vi "Accurate Measure With Setting_ver2_2.vi"(0 "DMM ref in":refnum<visa-resource-name>, 1 "Accurate Measure Setting":T1={"Enable DMM Relay"=FALSE, "Measure Current Only"=FALSE, [], "channel_count"=11}, 2 "P_current_count":i32, 3 "N_current_count":i32, 5 "DMM error in":errorcluster, 7 "Current Sense \nResitance Array":dbl[](array[numeric])=[1.0032214, 1.00250644, 1.00234822, 1.0040944, 1.0017711, 1.00229431, 1.00344206, 1.00482066, 1.00381056, 1.00290978, 1.00333016, 1.00367587], 9 "ESP32 ref in":refnum<visa-resource-name>, 11 "ESP32 error in":errorcluster, 12 "current_mode":u8[](array[numeric])=[0, 0, 0, 0, 0, 0, 0, 0, 0, 0, 0]) -> (4 "DMM ref out":refnum<visa-resource-name>, 6 "DMM error out":errorcluster, 8 "Accurate Data":dbl[](array[numeric]), 10 "ESP32 ref out":refnum<visa-resource-name>, 13 "time_out_count":i32, 14 "Standard Deviation of Data":dbl[](array[numeric]), 15 "ESP32 error out":errorcluster)   [LabVIEW 2023]
uses:
  <instrlib>/Agilent 3446X Series/Agilent 3446X Series.lvlib
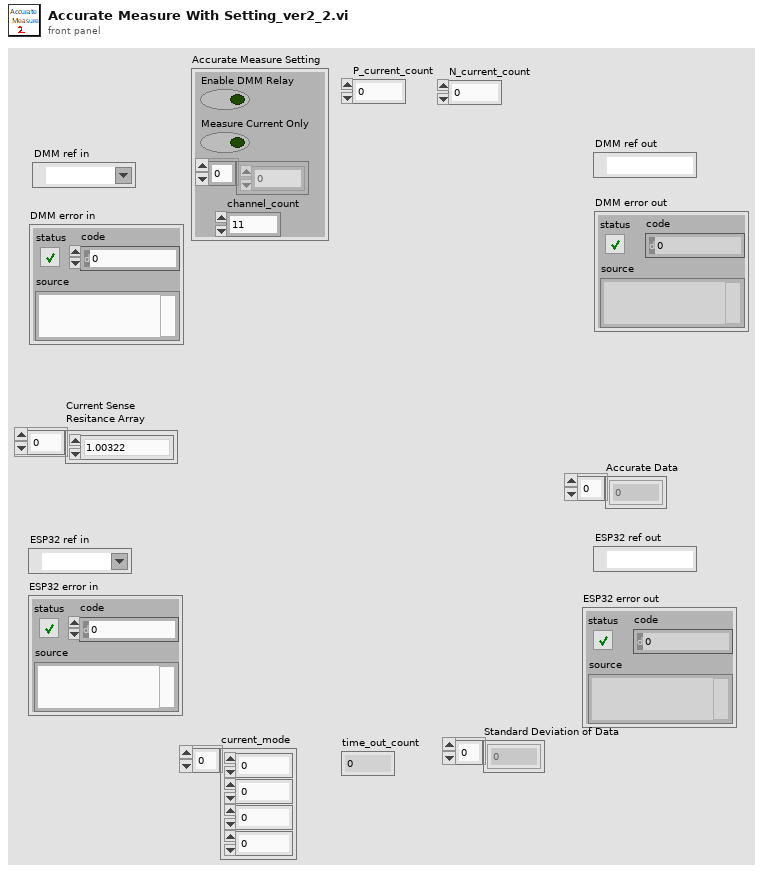
[diagram p1: front panel]
types:
  T1 = cluster{"Enable DMM Relay":bool, "Measure Current Only":bool, dbl[], "channel_count":i32}
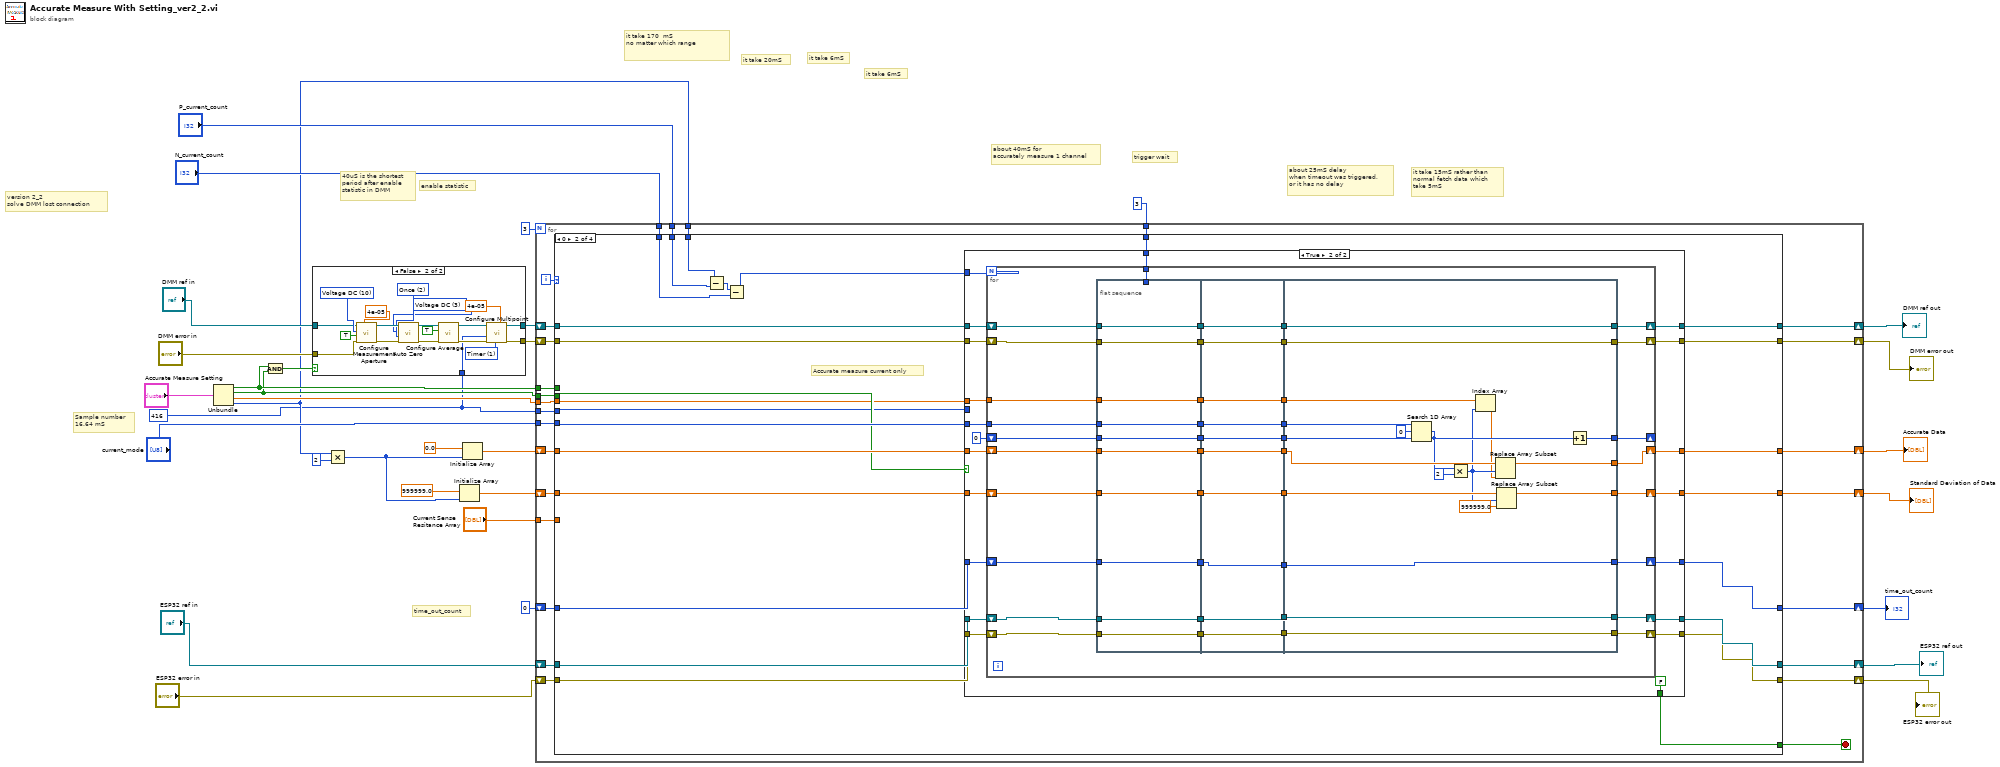
[diagram p0: block diagram]
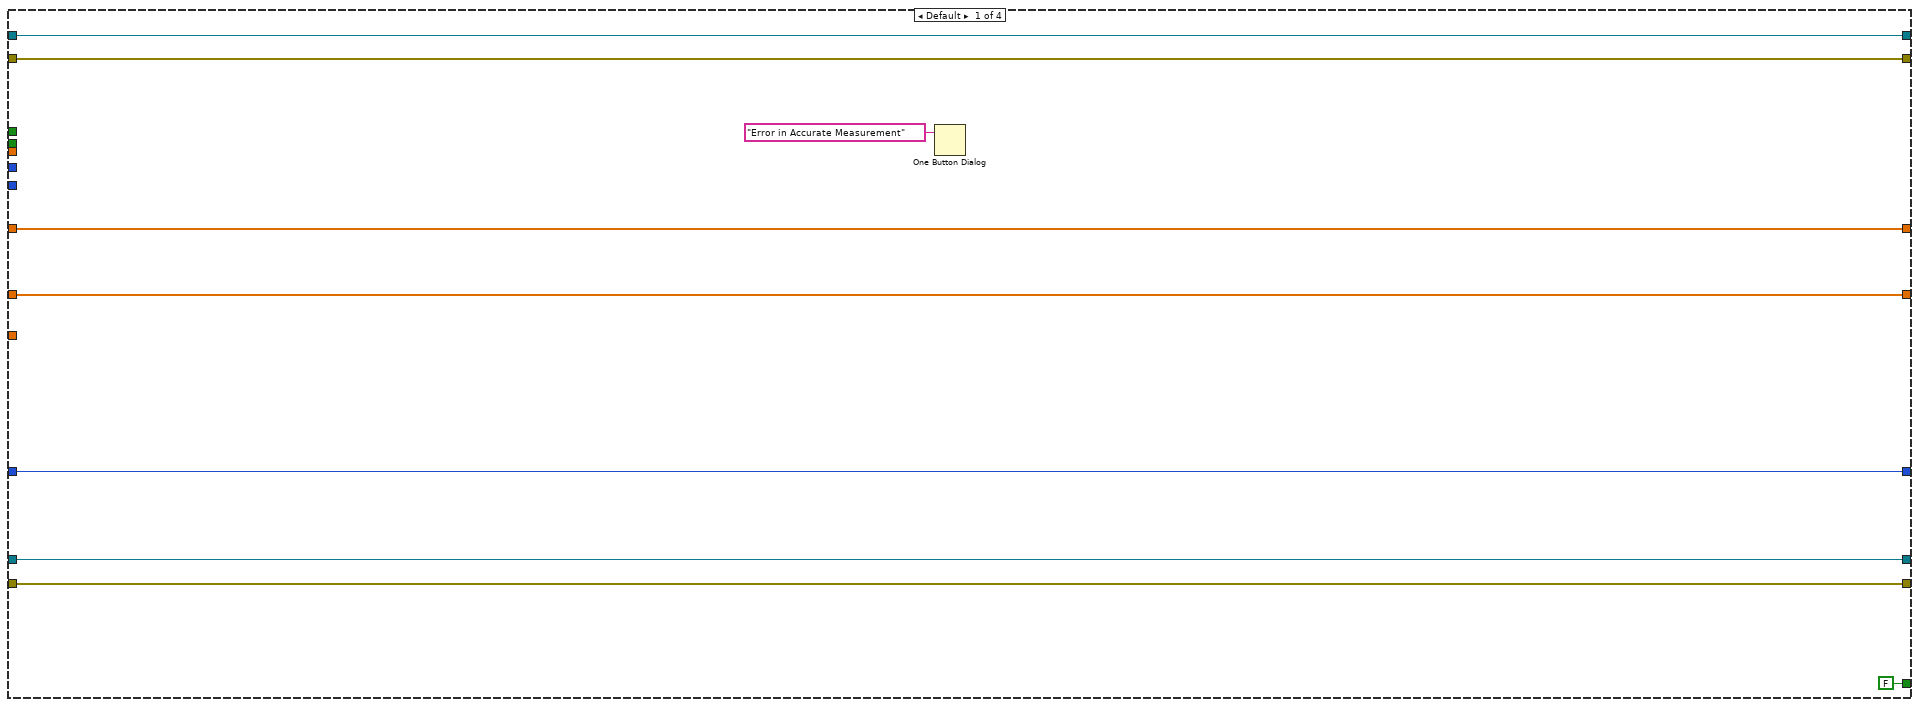
[diagram p3: hidden frame]
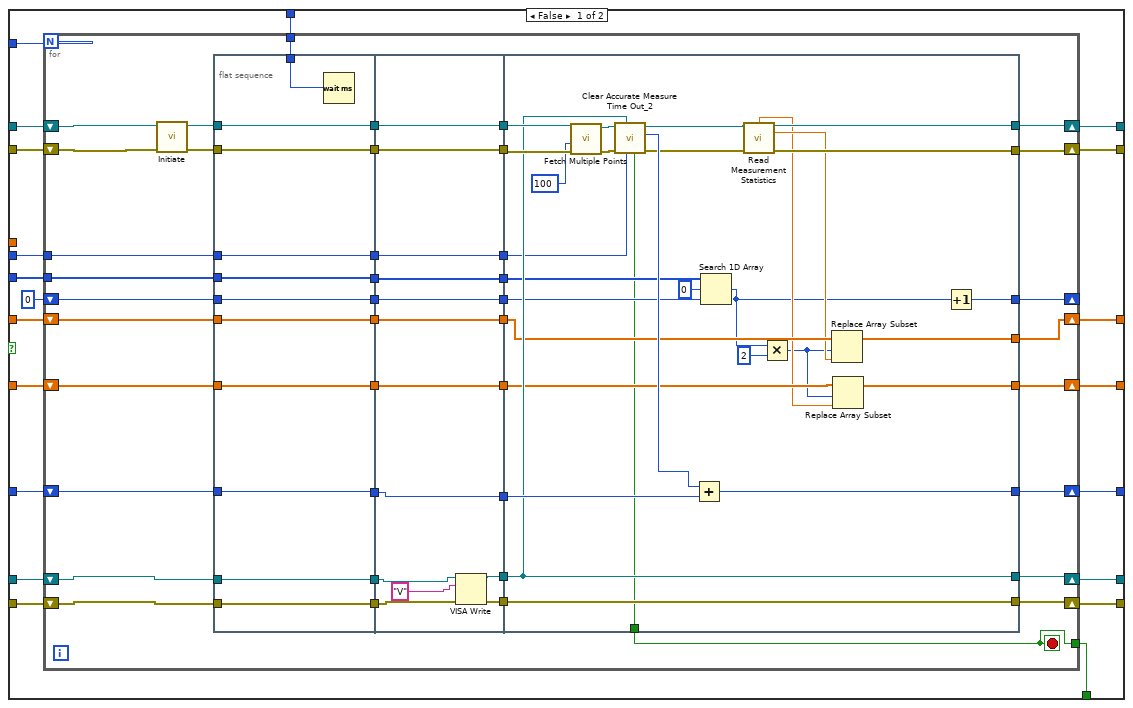
[diagram p4: hidden frame]
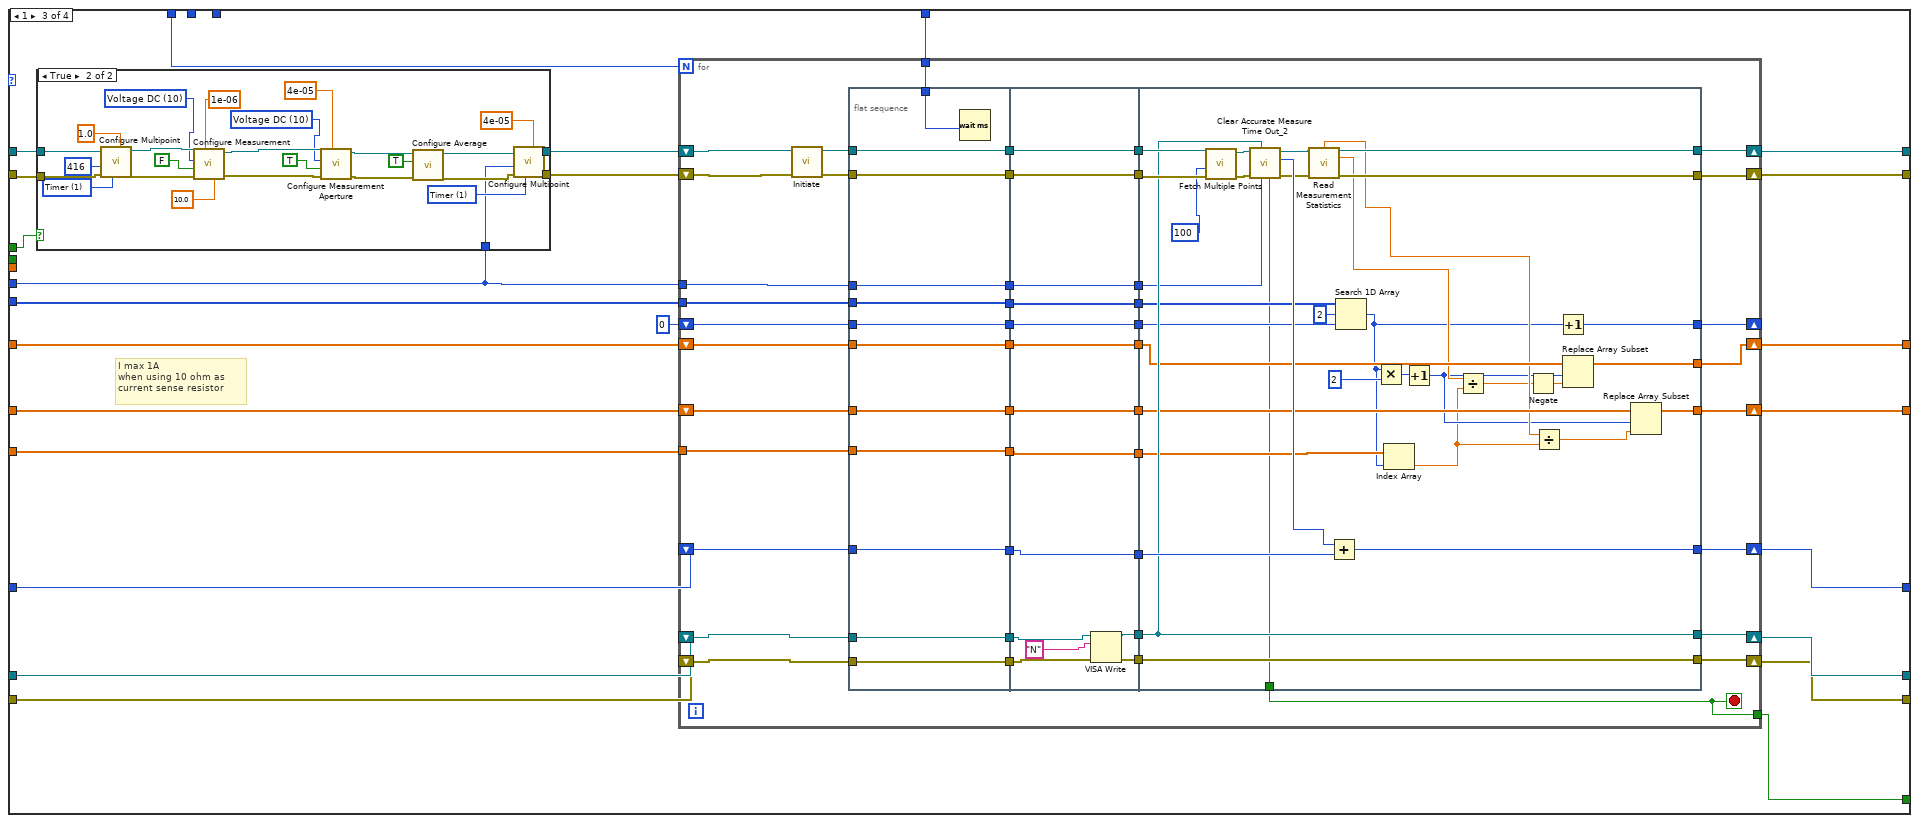
[diagram p5: hidden frame]
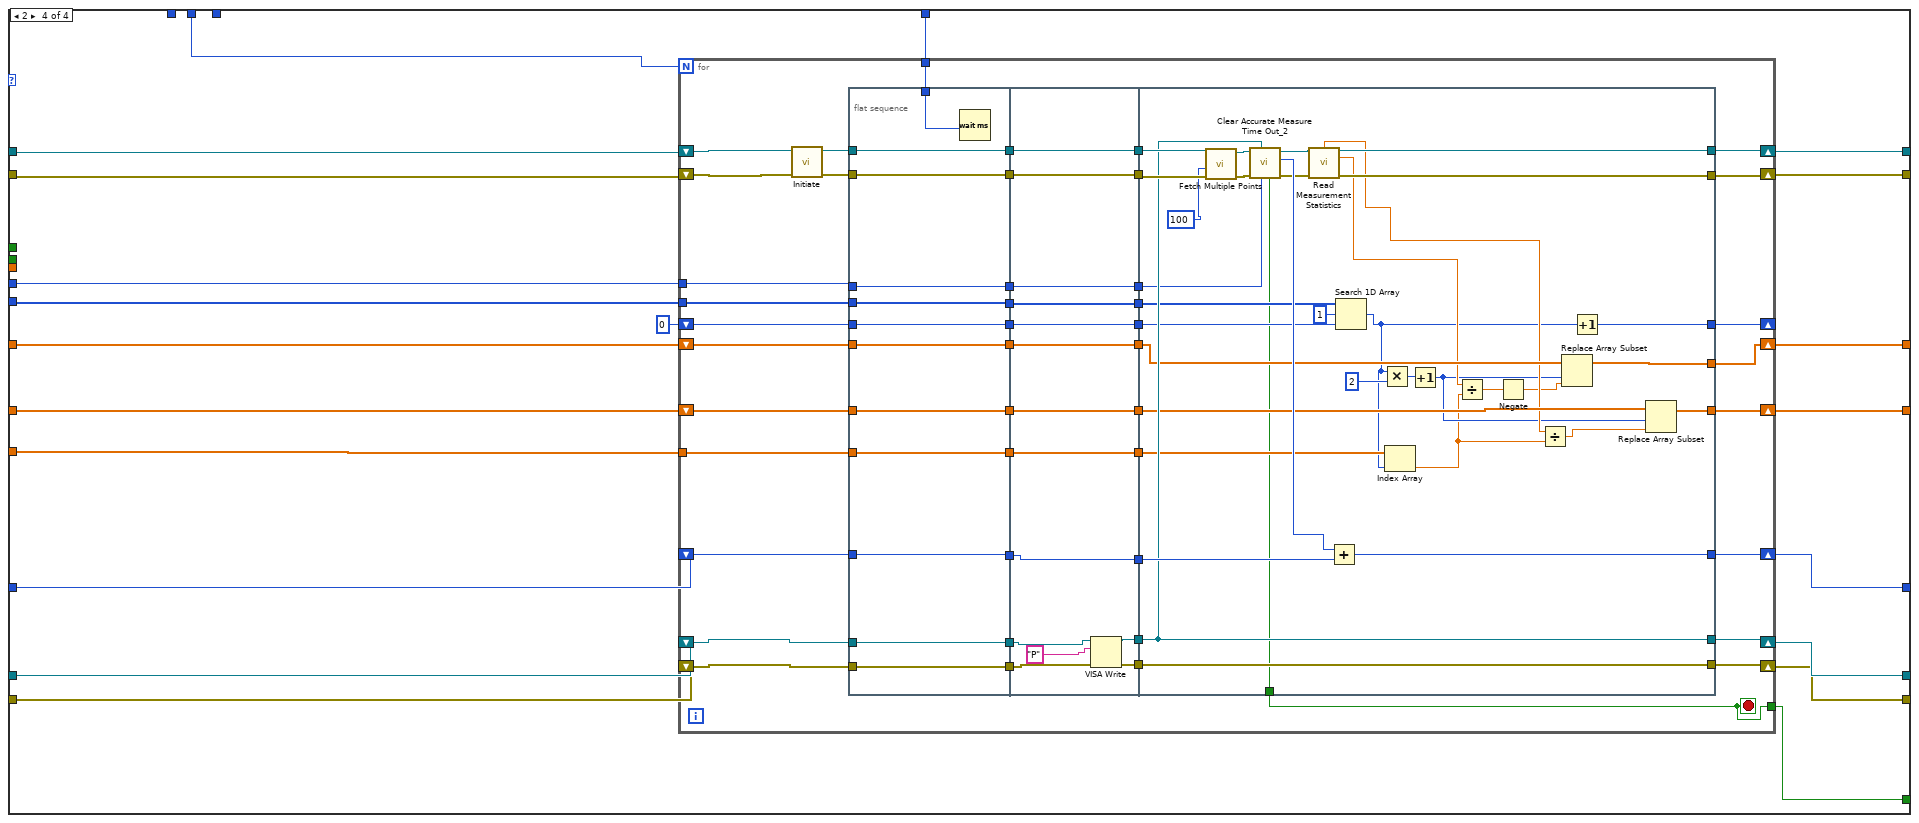
[diagram p7: hidden frame]
diagram:
  w1 = 416 ("Sample Count (1)")
  # "version 2_2\nsolve DMM lost connection"
  # "it take 6mS"
  # "it take 6mS"
  # "it take 20mS"
  # "it take 170  mS\nno matter which range"
  # "it take 15mS rather than\nnormal fetch data which \ntake 5mS"
  # "about 40mS for \naccurately measure 1 channel"
  # "about 25mS delay\nwhen timeout was triggered,\nor it has no delay"
  # "time_out_count"
  # "trigger wait"
  # "Sample number\n16.64 mS"
  # "enable statistic"
  # "40uS is the shortest\nperiod after enable \nstatistic in DMM"
  n1 = Unbundle("Accurate Measure Setting") -> ("Enable DMM Relay"=w6:bool, "Measure Current Only"=w5:bool, w7:dbl[], "channel_count"=w3:i32)
  n2 = And(x=w6, y=w5) -> (x .and. y?=w4:bool)
  n3 = case shown="False" w4 {
    tunnel: [w35 w40] -> w33
    tunnel: [w34 w39] -> w32
    tunnel: "DMM ref in" -> [w35 w38]
    tunnel: "DMM error in" -> [w34 w37]
    tunnel: w1 -> [_ w36]
    frame True {
    }
    frame False {
      w41 = 1 items=["Immediate", "Timer"] ("Sample Source (0: Immediate)")
      w48 = 3 items=["Current DC", "Resistance", "Temperature", "Voltage DC"] ("Zero Type (0: Current DC)")
      w49 = 2 items=["Disable", "Enable", "Once"] ("Auto Zero (1: Enable)")
      w45 = 10 items=["Continuity", "Current AC", "Current DC", "Diode", "Frequency", "Resistance 4-wire", "Period", "Resistance 2-wire", "Temperature", "Voltage AC", "Voltage DC", "Voltage DC Ratio", "Capacitance"] ("Measurement Function (0: Continuity)")
      n4 = call <instrlib>:"Configure Measurement Aperture.vi"("Aperture Time (0.1s)"=4e-05, "error in (no error)"=w37, "Enable Aperture (F: Disable)"=TRUE, "Measurement Function (0: Continuity)"=w45, "VISA resource name"=w38) -> ("error out"=w52:errorcluster, "VISA resource name out"=w51:refnum<visa-resource-name>)  [unwired: 5 in]
      n5 = call <instrlib>:"Auto Zero.vi"("error in (no error)"=w52, "Auto Zero (1: Enable)"=w49, "Zero Type (0: Current DC)"=w48, "VISA resource name"=w51) -> ("error out"=w54:errorcluster, "VISA resource name out"=w53:refnum<visa-resource-name>)  [unwired: 6 in]
      n6 = call <instrlib>:"Configure Average.vi"("error in (no error)"=w54, "Enable Statistics (F: Disable)"=TRUE, "VISA resource name"=w53) -> ("error out"=w43:errorcluster, "VISA resource name out"=w44:refnum<visa-resource-name>)  [unwired: 7 in]
      n7 = call <instrlib>:"Configure Multipoint.vi"("Sample Interval (1 Second)"=4e-05, "Sample Source (0: Immediate)"=w41, "error in (no error)"=w43, "Sample Count (1)"=w36, "VISA resource name"=w44) -> ("error out"=w39:errorcluster, "VISA resource name out"=w40:refnum<visa-resource-name>)  [unwired: 2 in, 3 out]
    }
  }
  n8 = Multiply(x=w3, y=2) -> (x*y=w9:i32)
  n9 = Initialize Array(999999.0 ("Arithmetic Mean"), w9) -> (w18:dbl[])
  n10 = Initialize Array(0.0 ("Arithmetic Mean"), w9) -> (w21:dbl[])
  n11 = for {
    N: 3 -> [_]
    shift-right: [w78] -> w14
    shift-left: "ESP32 ref in" -> [w80]
    shift-right: [w77] -> w13
    shift-left: "ESP32 error in" -> [w79]
    shift-right: [w74] -> w16
    shift-left: w33 -> [w76]
    shift-right: [w73] -> w15
    shift-left: w32 -> [w75]
    tunnel: w3 -> [w72]
    tunnel: "P_current_count" -> [w71]
    tunnel: "N_current_count" -> [w70]
    tunnel: u32 3 ("milliseconds to wait") -> [w69]
    shift-right: [w68] -> w23
    shift-left: 0 -> [w67]
    shift-right: [w61] -> w12
    shift-left: w21 -> [w66]
    tunnel: "current_mode" -> [w65]
    shift-right: [w62] -> w11
    shift-left: w18 -> [w63]
    tunnel: w6 -> [w60]
    tunnel: w5 -> [w59]
    tunnel: w7 -> [w58]
    tunnel: "Current Sense \nResitance Array" -> [w57]
    tunnel: w1 -> [w56]
    i -> [w64]
    stop <- w55 stop-if-true
    n12 = case shown="0" w64 {
      tunnel: w80 -> [w87 w110 w351 w506]
      tunnel: w79 -> [w86 w109 w350 w505]
      tunnel: [w87 w106 w347 w502] -> w78
      tunnel: [w86 w105 w346 w501] -> w77
      tunnel: w76 -> [w89 w112 w336 w491]
      tunnel: w75 -> [w88 w111 w335 w490]
      tunnel: [w89 w108 w349 w504] -> w74
      tunnel: [w88 w107 w348 w503] -> w73
      tunnel: w72 -> [_ w104 _ _]
      tunnel: w71 -> [_ w103 _ w488]
      tunnel: w70 -> [_ w102 w330 _]
      tunnel: [w83 w100 w344 w499] -> w68
      tunnel: w69 -> [_ w101 w345 w500]
      tunnel: w67 -> [w83 w99 w343 w498]
      tunnel: w66 -> [w85 w97 w341 w496]
      tunnel: w65 -> [_ w98 w342 w497]
      tunnel: w63 -> [w84 w96 w339 w494]
      tunnel: [w84 w95 w338 w493] -> w62
      tunnel: [w85 w94 w337 w492] -> w61
      tunnel: w60 -> [_ _ w332 _]
      tunnel: w59 -> [_ w93 _ _]
      tunnel: w58 -> [_ w92 _ _]
      tunnel: w57 -> [_ _ w331 w489]
      tunnel: w56 -> [_ w91 w329 w487]
      tunnel: [FALSE ("lost connection") w90 w328 w486] -> w55
      frame Default {
        n13 = One Button Dialog(message="Error in Accurate Measurement") -> ()  [unwired: 1 in, 1 out]
      }
      frame 0 {
        # "Accurate measure current only"
        n14 = Subtract(x=w104, y=w103) -> (x-y=w114:i32)
        n15 = Subtract(x=w114, y=w102) -> (x-y=w113:i32)
        n16 = case shown="True" w93 {
          tunnel: w113 -> [w134 w249]
          tunnel: w112 -> [w133 w248]
          tunnel: w111 -> [w132 w247]
          tunnel: w110 -> [w131 w246]
          tunnel: w109 -> [w130 w245]
          tunnel: [w129 w244] -> w108
          tunnel: [w128 w243] -> w107
          tunnel: [w127 w242] -> w106
          tunnel: [w126 w241] -> w105
          tunnel: w101 -> [w125 w240]
          tunnel: [w124 w239] -> w100
          tunnel: w99 -> [w123 w238]
          tunnel: w98 -> [w122 w237]
          tunnel: w97 -> [w121 w236]
          tunnel: w96 -> [w119 w234]
          tunnel: [w118 w233] -> w95
          tunnel: [w117 w232] -> w94
          tunnel: w92 -> [_ w231]
          tunnel: w91 -> [w116 _]
          tunnel: [w115 FALSE ("lost connection")] -> w90
          frame False {
            n17 = for {
              N: w134 -> [_]
              shift-right: [w172] -> w129
              shift-left: w133 -> [w176]
              shift-right: [w171] -> w128
              shift-left: w132 -> [w175]
              shift-right: [w170] -> w127
              shift-left: w131 -> [w174]
              shift-right: [w169] -> w126
              shift-left: w130 -> [w173]
              tunnel: w125 -> [w155]
              shift-right: [w154] -> w124
              shift-left: w123 -> [w168]
              tunnel: w122 -> [w152]
              shift-right: [w140] -> w117
              shift-left: w121 -> [w149]
              shift-right: [w144] -> _
              shift-left: 0 ("index of element") -> [w145]
              shift-right: [w139] -> w118
              shift-left: w119 -> [w142]
              tunnel: w116 -> [w136]
              tunnel: [w135] -> w115
              stop <- w135 stop-if-true
              n18 = call <instrlib>:"Initiate.vi"("error in (no error)"=w175, "VISA resource name"=w176) -> ("error out"=w156:errorcluster, "VISA resource name out"=w157:refnum<visa-resource-name>)  [unwired: 8 in]
              n19 = flat-sequence {
                tunnel: [w187] -> w167
                tunnel: w174 -> [w187]
                tunnel: [w186] -> w166
                tunnel: w173 -> [w186]
                tunnel: w157 -> [w185]
                tunnel: [w185] -> w165
                tunnel: [w184] -> w164
                tunnel: w156 -> [w184]
                tunnel: [w183] -> w163
                tunnel: w168 -> [w183]
                tunnel: w155 -> [w182]
                tunnel: [w181] -> w153
                tunnel: w152 -> [w181]
                tunnel: [w180] -> w150
                tunnel: w149 -> [w180]
                tunnel: w145 -> [w179]
                tunnel: [w179] -> w147
                tunnel: [w178] -> w143
                tunnel: w142 -> [w178]
                tunnel: w136 -> [w177]
                tunnel: [w177] -> w138
                tunnel: w167 -> [w200]
                tunnel: w166 -> [w199]
                tunnel: w165 -> [w198]
                tunnel: [w198] -> w159
                tunnel: w164 -> [w197]
                tunnel: [w197] -> w160
                tunnel: [w196] -> w161
                tunnel: [w195] -> w162
                tunnel: w163 -> [w193]
                tunnel: [w193] -> w158
                tunnel: w153 -> [w192]
                tunnel: [w192] -> w151
                tunnel: w150 -> [w191]
                tunnel: [w191] -> w148
                tunnel: w147 -> [w190]
                tunnel: [w190] -> w146
                tunnel: w143 -> [w189]
                tunnel: [w189] -> w141
                tunnel: w138 -> [w188]
                tunnel: [w188] -> w137
                tunnel: [w229] -> w169
                tunnel: [w217] -> w170
                tunnel: [w221] -> w171
                tunnel: [w222] -> w172
                tunnel: w162 -> [w229]
                tunnel: w161 -> [w217]
                tunnel: w160 -> [w228]
                tunnel: w159 -> [w227]
                tunnel: [w223] -> w154
                tunnel: w158 -> [w218]
                tunnel: w151 -> [w216]
                tunnel: w148 -> [w212]
                tunnel: w146 -> [w214]
                tunnel: [w213] -> w144
                tunnel: w141 -> [w210]
                tunnel: [w208] -> w140
                tunnel: [w207] -> w139
                tunnel: w137 -> [w202]
                tunnel: [w201] -> w135
                frame #0 {
                  n20 = Wait (ms)(milliseconds to wait=w182) -> ()  [unwired: 1 out]
                }
                frame #1 {
                  n21 = VISA Write(VISA resource name=w200, write buffer="V" ("data in"), error in (no error)=w199) -> (VISA resource name out=w196:refnum<visa-resource-name>, error out=w195:errorcluster)  [unwired: 1 out]
                }
                frame #2 {
                  n22 = call <instrlib>:"Fetch Multiple Points.vi"("error in (no error)"=w228, "Timeout (10000 ms)"=100, "VISA resource name"=w227) -> ("error out"=w225:errorcluster, "VISA resource name out"=w226:refnum<visa-resource-name>)  [unwired: 1 in, 6 out]
                  n23 = call "Clear Accurate Measure Time Out_2.vi"("Sample Count (1)"=w202, "ESP32 ref"=w217, "error in (no error)"=w225, "DMM ref"=w226) -> ("error out"=w219:errorcluster, "Time out count"=w224:i32, "VISA Refnum out"=w220:refnum<visa-resource-name>, "lost connection"=w201:bool)  [unwired: 3 in, 1 out]
                  n24 = Add(x=w224, y=w218) -> (x+y=w223:i32)
                  n25 = Search 1D Array(1D array=w216, element=u8 0, start index (0)=w214) -> (index of element=w205:i32)
                  n26 = call <instrlib>:"Read Measurement Statistics.vi"("VISA resource name"=w220, "error in (no error)"=w219) -> ("Standard Deviation"=w209:dbl, "VISA resource name out"=w222:refnum<visa-resource-name>, "Arithmetic Mean"=w211:dbl, "error out"=w221:errorcluster)  [unwired: 6 in, 4 out]
                  n27 = Multiply(x=w205, y=2) -> (x*y=w203:i32)
                  n28 = Replace Array Subset(array=w212, new element=w211, index=w203) -> (w208:dbl[])
                  n29 = Replace Array Subset(array=w210, new element=w209, index=w203) -> (w207:dbl[])
                  n30 = Increment(x=w205) -> (x+1=w213:i32)
                }
              }
            }
          }
          frame True {
            n31 = for {
              N: w249 -> [_]
              shift-right: [w258] -> w244
              shift-left: w248 -> [w260]
              shift-right: [w253] -> w243
              shift-left: w247 -> [w255]
              shift-right: [w286] -> w242
              shift-left: w246 -> [w288]
              shift-right: [w285] -> w241
              shift-left: w245 -> [w287]
              tunnel: w240 -> [w277]
              shift-right: [w276] -> w239
              shift-left: w238 -> [w284]
              tunnel: w237 -> [w274]
              shift-right: [w262] -> w232
              shift-left: w236 -> [w271]
              shift-right: [w266] -> _
              shift-left: 0 ("index of element") -> [w267]
              shift-right: [w261] -> w233
              shift-left: w234 -> [w264]
              tunnel: w231 -> [w250]
              n32 = flat-sequence {
                tunnel: [w298] -> w283
                tunnel: w288 -> [w298]
                tunnel: [w297] -> w282
                tunnel: w287 -> [w297]
                tunnel: [w296] -> w281
                tunnel: w284 -> [w296]
                tunnel: w277 -> [_]
                tunnel: [w295] -> w275
                tunnel: w274 -> [w295]
                tunnel: [w294] -> w272
                tunnel: w271 -> [w294]
                tunnel: w267 -> [w293]
                tunnel: [w293] -> w269
                tunnel: [w292] -> w265
                tunnel: w264 -> [w292]
                tunnel: w260 -> [w291]
                tunnel: [w291] -> w257
                tunnel: [w290] -> w256
                tunnel: w255 -> [w290]
                tunnel: [w289] -> w252
                tunnel: w250 -> [w289]
                tunnel: w283 -> [w301]
                tunnel: w282 -> [w300]
                tunnel: [w301] -> w279
                tunnel: [w300] -> w280
                tunnel: w281 -> [w308]
                tunnel: [w308] -> w278
                tunnel: w275 -> [w307]
                tunnel: [w307] -> w273
                tunnel: w272 -> [w306]
                tunnel: [w306] -> w270
                tunnel: w269 -> [w305]
                tunnel: [w305] -> w268
                tunnel: w265 -> [w304]
                tunnel: [w304] -> w263
                tunnel: [w303] -> w259
                tunnel: w257 -> [w303]
                tunnel: w256 -> [w302]
                tunnel: [w302] -> w254
                tunnel: w252 -> [w299]
                tunnel: [w299] -> w251
                tunnel: [w327] -> w285
                tunnel: [w326] -> w286
                tunnel: w280 -> [w327]
                tunnel: w279 -> [w326]
                tunnel: [w309] -> w276
                tunnel: w278 -> [w309]
                tunnel: w273 -> [w325]
                tunnel: w270 -> [w321]
                tunnel: w268 -> [w323]
                tunnel: [w322] -> w266
                tunnel: w263 -> [w320]
                tunnel: [w319] -> w262
                tunnel: [w318] -> w261
                tunnel: w259 -> [w315]
                tunnel: [w315] -> w258
                tunnel: [w314] -> w253
                tunnel: w254 -> [w314]
                tunnel: w251 -> [w312]
                frame #0 {
                }
                frame #1 {
                }
                frame #2 {
                  n33 = Search 1D Array(1D array=w325, element=u8 0, start index (0)=w323) -> (index of element=w317:i32)
                  n34 = Multiply(x=w317, y=2) -> (x*y=w311:i32)
                  n35 = Index Array(array=w312, index=w311) -> (element=w310:dbl)
                  n36 = Replace Array Subset(array=w321, new element=w310, index=w311) -> (w319:dbl[])
                  n37 = Replace Array Subset(array=w320, new element=999999.0 ("new element/subarray"), index=w311) -> (w318:dbl[])
                  n38 = Increment(x=w317) -> (x+1=w322:i32)
                }
              }
            }
          }
        }
      }
      frame 1 {
        # "I max 1A\nwhen using 10 ohm as \ncurrent sense resistor"
        n39 = case shown="True" w332 {
          tunnel: w336 -> [w353 w360]
          tunnel: w335 -> [w352 w359]
          tunnel: [w353 w358] -> w334
          tunnel: [w352 w357] -> w333
          tunnel: w329 -> [_ w354]
          frame False {
          }
          frame True {
            w369 = 1 items=["Immediate", "Timer"] ("Sample Source (0: Immediate)")
            w366 = 10 items=["Continuity", "Current AC", "Current DC", "Diode", "Frequency", "Resistance 4-wire", "Period", "Resistance 2-wire", "Temperature", "Voltage AC", "Voltage DC", "Voltage DC Ratio", "Capacitance"] ("Measurement Function (0: Continuity)")
            w364 = 1 items=["Immediate", "Timer"] ("Sample Source (0: Immediate)")
            w361 = 10 items=["Continuity", "Current AC", "Current DC", "Diode", "Frequency", "Resistance 4-wire", "Period", "Resistance 2-wire", "Temperature", "Voltage AC", "Voltage DC", "Voltage DC Ratio", "Capacitance"] ("Measurement Function (10: Voltage DC)")
            n40 = call <instrlib>:"Configure Multipoint.vi"("Sample Interval (1 Second)"=1.0, "Sample Source (0: Immediate)"=w364, "error in (no error)"=w359, "Sample Count (1)"=416, "VISA resource name"=w360) -> ("error out"=w376:errorcluster, "VISA resource name out"=w375:refnum<visa-resource-name>)  [unwired: 2 in, 3 out]
            n41 = call <instrlib>:"Configure Measurement.vi"("Manual Range (1)"=10.0, "Absolute Resolution (1E-6)"=1e-06 ("x"), "error in (no error)"=w376, "Auto Range (T: Enable)"=FALSE, "Measurement Function (10: Voltage DC)"=w361, "VISA resource name"=w375) -> ("error out"=w373:errorcluster, "VISA resource name out"=w374:refnum<visa-resource-name>)  [unwired: 4 out]
            n42 = call <instrlib>:"Configure Measurement Aperture.vi"("Aperture Time (0.1s)"=4e-05, "error in (no error)"=w373, "Enable Aperture (F: Disable)"=TRUE, "Measurement Function (0: Continuity)"=w366, "VISA resource name"=w374) -> ("error out"=w378:errorcluster, "VISA resource name out"=w379:refnum<visa-resource-name>)  [unwired: 5 in]
            n43 = call <instrlib>:"Configure Average.vi"("error in (no error)"=w378, "Enable Statistics (F: Disable)"=TRUE, "VISA resource name"=w379) -> ("error out"=w377:errorcluster, "VISA resource name out"=w372:refnum<visa-resource-name>)  [unwired: 7 in]
            n44 = call <instrlib>:"Configure Multipoint.vi"("Sample Interval (1 Second)"=4e-05, "Sample Source (0: Immediate)"=w369, "error in (no error)"=w377, "Sample Count (1)"=w354, "VISA resource name"=w372) -> ("error out"=w357:errorcluster, "VISA resource name out"=w358:refnum<visa-resource-name>)  [unwired: 2 in, 3 out]
          }
        }
        n45 = for {
          N: w330 -> [_]
          shift-right: [w420] -> w349
          shift-left: w334 -> [w424]
          shift-right: [w419] -> w348
          shift-left: w333 -> [w423]
          shift-right: [w418] -> w347
          shift-left: w351 -> [w422]
          shift-right: [w417] -> w346
          shift-left: w350 -> [w421]
          tunnel: w345 -> [w403]
          shift-right: [w402] -> w344
          shift-left: w343 -> [w416]
          tunnel: w342 -> [w400]
          shift-right: [w388] -> w337
          shift-left: w341 -> [w397]
          shift-right: [w392] -> _
          shift-left: 0 ("index of element") -> [w393]
          shift-right: [w387] -> w338
          shift-left: w339 -> [w390]
          tunnel: w331 -> [w385]
          tunnel: w329 -> [w383]
          tunnel: [w380] -> w328
          stop <- w380 stop-if-true
          n46 = call <instrlib>:"Initiate.vi"("error in (no error)"=w423, "VISA resource name"=w424) -> ("error out"=w404:errorcluster, "VISA resource name out"=w405:refnum<visa-resource-name>)  [unwired: 8 in]
          n47 = flat-sequence {
            tunnel: [w436] -> w415
            tunnel: w422 -> [w436]
            tunnel: [w435] -> w414
            tunnel: w421 -> [w435]
            tunnel: w405 -> [w434]
            tunnel: [w434] -> w413
            tunnel: [w433] -> w412
            tunnel: w404 -> [w433]
            tunnel: [w432] -> w411
            tunnel: w416 -> [w432]
            tunnel: w403 -> [w431]
            tunnel: [w430] -> w401
            tunnel: w400 -> [w430]
            tunnel: [w429] -> w398
            tunnel: w397 -> [w429]
            tunnel: w393 -> [w428]
            tunnel: [w428] -> w395
            tunnel: [w427] -> w391
            tunnel: w390 -> [w427]
            tunnel: [w426] -> w386
            tunnel: w385 -> [w426]
            tunnel: w383 -> [w425]
            tunnel: [w425] -> w382
            tunnel: w415 -> [w450]
            tunnel: w414 -> [w449]
            tunnel: w413 -> [w448]
            tunnel: [w448] -> w407
            tunnel: w412 -> [w447]
            tunnel: [w447] -> w408
            tunnel: [w446] -> w409
            tunnel: [w445] -> w410
            tunnel: w411 -> [w443]
            tunnel: [w443] -> w406
            tunnel: w401 -> [w442]
            tunnel: [w442] -> w399
            tunnel: w398 -> [w441]
            tunnel: [w441] -> w396
            tunnel: w395 -> [w440]
            tunnel: [w440] -> w394
            tunnel: w391 -> [w439]
            tunnel: [w439] -> w389
            tunnel: w386 -> [w438]
            tunnel: [w438] -> w384
            tunnel: w382 -> [w437]
            tunnel: [w437] -> w381
            tunnel: [w485] -> w417
            tunnel: [w473] -> w418
            tunnel: [w477] -> w419
            tunnel: [w478] -> w420
            tunnel: w410 -> [w485]
            tunnel: w409 -> [w473]
            tunnel: w408 -> [w484]
            tunnel: w407 -> [w483]
            tunnel: [w479] -> w402
            tunnel: w406 -> [w474]
            tunnel: w399 -> [w472]
            tunnel: w396 -> [w469]
            tunnel: w394 -> [w471]
            tunnel: [w470] -> w392
            tunnel: w389 -> [w468]
            tunnel: [w467] -> w388
            tunnel: [w466] -> w387
            tunnel: w384 -> [w462]
            tunnel: w381 -> [w452]
            tunnel: [w451] -> w380
            frame #0 {
              n48 = Wait (ms)(milliseconds to wait=w431) -> ()  [unwired: 1 out]
            }
            frame #1 {
              n49 = VISA Write(VISA resource name=w450, write buffer="N" ("data in"), error in (no error)=w449) -> (VISA resource name out=w446:refnum<visa-resource-name>, error out=w445:errorcluster)  [unwired: 1 out]
            }
            frame #2 {
              n50 = call <instrlib>:"Fetch Multiple Points.vi"("error in (no error)"=w484, "Timeout (10000 ms)"=100, "VISA resource name"=w483) -> ("error out"=w481:errorcluster, "VISA resource name out"=w482:refnum<visa-resource-name>)  [unwired: 1 in, 6 out]
              n51 = call "Clear Accurate Measure Time Out_2.vi"("Sample Count (1)"=w452, "ESP32 ref"=w473, "error in (no error)"=w481, "DMM ref"=w482) -> ("error out"=w475:errorcluster, "Time out count"=w480:i32, "VISA Refnum out"=w476:refnum<visa-resource-name>, "lost connection"=w451:bool)  [unwired: 3 in, 1 out]
              n52 = call <instrlib>:"Read Measurement Statistics.vi"("VISA resource name"=w476, "error in (no error)"=w475) -> ("Standard Deviation"=w464:dbl, "VISA resource name out"=w478:refnum<visa-resource-name>, "Arithmetic Mean"=w465:dbl, "error out"=w477:errorcluster)  [unwired: 6 in, 4 out]
              n53 = Add(x=w480, y=w474) -> (x+y=w479:i32)
              n54 = Search 1D Array(1D array=w472, element=u8 2, start index (0)=w471) -> (index of element=w457:i32)
              n55 = Multiply(x=w457, y=2) -> (x*y=w459:i32)
              n56 = Index Array(array=w462, index=w457) -> (element=w455:dbl)
              n57 = Increment(x=w459) -> (x+1=w458:i32)
              n58 = Divide(x=w465, y=w455) -> (x/y=w456:dbl)
              n59 = Negate(x=w456) -> (-x=w453:dbl)
              n60 = Divide(x=w464, y=w455) -> (x/y=w454:dbl)
              n61 = Increment(x=w457) -> (x+1=w470:i32)
              n62 = Replace Array Subset(array=w469, new element=w453, index=w458) -> (w467:dbl[])
              n63 = Replace Array Subset(array=w468, new element=w454, index=w458) -> (w466:dbl[])
            }
          }
        }
      }
      frame 2 {
        n64 = for {
          N: w488 -> [_]
          shift-right: [w547] -> w504
          shift-left: w491 -> [w551]
          shift-right: [w546] -> w503
          shift-left: w490 -> [w550]
          shift-right: [w545] -> w502
          shift-left: w506 -> [w549]
          shift-right: [w544] -> w501
          shift-left: w505 -> [w548]
          tunnel: w500 -> [w530]
          shift-right: [w529] -> w499
          shift-left: w498 -> [w543]
          tunnel: w497 -> [w527]
          shift-right: [w515] -> w492
          shift-left: w496 -> [w524]
          shift-right: [w519] -> _
          shift-left: 0 ("index of element") -> [w520]
          shift-right: [w514] -> w493
          shift-left: w494 -> [w517]
          tunnel: w489 -> [w512]
          tunnel: w487 -> [w508]
          tunnel: [w507] -> w486
          stop <- w507 stop-if-true
          n65 = call <instrlib>:"Initiate.vi"("error in (no error)"=w550, "VISA resource name"=w551) -> ("error out"=w531:errorcluster, "VISA resource name out"=w532:refnum<visa-resource-name>)  [unwired: 8 in]
          n66 = flat-sequence {
            tunnel: [w563] -> w542
            tunnel: w549 -> [w563]
            tunnel: [w562] -> w541
            tunnel: w548 -> [w562]
            tunnel: w532 -> [w561]
            tunnel: [w561] -> w540
            tunnel: [w560] -> w539
            tunnel: w531 -> [w560]
            tunnel: [w559] -> w538
            tunnel: w543 -> [w559]
            tunnel: w530 -> [w558]
            tunnel: [w557] -> w528
            tunnel: w527 -> [w557]
            tunnel: [w556] -> w525
            tunnel: w524 -> [w556]
            tunnel: w520 -> [w555]
            tunnel: [w555] -> w522
            tunnel: [w554] -> w518
            tunnel: w517 -> [w554]
            tunnel: [w553] -> w513
            tunnel: w512 -> [w553]
            tunnel: w508 -> [w552]
            tunnel: [w552] -> w510
            tunnel: w542 -> [w577]
            tunnel: w541 -> [w576]
            tunnel: w540 -> [w575]
            tunnel: [w575] -> w534
            tunnel: w539 -> [w574]
            tunnel: [w574] -> w535
            tunnel: [w573] -> w536
            tunnel: [w572] -> w537
            tunnel: w538 -> [w570]
            tunnel: [w570] -> w533
            tunnel: w528 -> [w569]
            tunnel: [w569] -> w526
            tunnel: w525 -> [w568]
            tunnel: [w568] -> w523
            tunnel: w522 -> [w567]
            tunnel: [w567] -> w521
            tunnel: w518 -> [w566]
            tunnel: [w566] -> w516
            tunnel: w513 -> [w565]
            tunnel: [w565] -> w511
            tunnel: w510 -> [w564]
            tunnel: [w564] -> w509
            tunnel: [w612] -> w544
            tunnel: [w600] -> w545
            tunnel: [w604] -> w546
            tunnel: [w605] -> w547
            tunnel: w537 -> [w612]
            tunnel: w536 -> [w600]
            tunnel: w535 -> [w611]
            tunnel: w534 -> [w610]
            tunnel: [w606] -> w529
            tunnel: w533 -> [w601]
            tunnel: w526 -> [w599]
            tunnel: w523 -> [w596]
            tunnel: w521 -> [w598]
            tunnel: [w597] -> w519
            tunnel: w516 -> [w595]
            tunnel: [w594] -> w515
            tunnel: [w593] -> w514
            tunnel: w511 -> [w589]
            tunnel: w509 -> [w579]
            tunnel: [w578] -> w507
            frame #0 {
              n67 = Wait (ms)(milliseconds to wait=w558) -> ()  [unwired: 1 out]
            }
            frame #1 {
              n68 = VISA Write(VISA resource name=w577, write buffer="P" ("data in"), error in (no error)=w576) -> (VISA resource name out=w573:refnum<visa-resource-name>, error out=w572:errorcluster)  [unwired: 1 out]
            }
            frame #2 {
              n69 = call <instrlib>:"Fetch Multiple Points.vi"("error in (no error)"=w611, "Timeout (10000 ms)"=100, "VISA resource name"=w610) -> ("error out"=w608:errorcluster, "VISA resource name out"=w609:refnum<visa-resource-name>)  [unwired: 1 in, 6 out]
              n70 = call "Clear Accurate Measure Time Out_2.vi"("Sample Count (1)"=w579, "ESP32 ref"=w600, "error in (no error)"=w608, "DMM ref"=w609) -> ("error out"=w602:errorcluster, "Time out count"=w607:i32, "VISA Refnum out"=w603:refnum<visa-resource-name>, "lost connection"=w578:bool)  [unwired: 3 in, 1 out]
              n71 = call <instrlib>:"Read Measurement Statistics.vi"("VISA resource name"=w603, "error in (no error)"=w602) -> ("Standard Deviation"=w591:dbl, "VISA resource name out"=w605:refnum<visa-resource-name>, "Arithmetic Mean"=w592:dbl, "error out"=w604:errorcluster)  [unwired: 6 in, 4 out]
              n72 = Add(x=w607, y=w601) -> (x+y=w606:i32)
              n73 = Search 1D Array(1D array=w599, element=u8 1, start index (0)=w598) -> (index of element=w584:i32)
              n74 = Multiply(x=w584, y=2) -> (x*y=w586:i32)
              n75 = Index Array(array=w589, index=w584) -> (element=w582:dbl)
              n76 = Increment(x=w586) -> (x+1=w585:i32)
              n77 = Divide(x=w592, y=w582) -> (x/y=w583:dbl)
              n78 = Negate(x=w583) -> (-x=w580:dbl)
              n79 = Divide(x=w591, y=w582) -> (x/y=w581:dbl)
              n80 = Replace Array Subset(array=w596, new element=w580, index=w585) -> (w594:dbl[])
              n81 = Increment(x=w584) -> (x+1=w597:i32)
              n82 = Replace Array Subset(array=w595, new element=w581, index=w585) -> (w593:dbl[])
            }
          }
        }
      }
    }
  }
  "time_out_count" <- w23
  "DMM ref out" <- w16
  "DMM error out" <- w15
  "ESP32 ref out" <- w14
  "ESP32 error out" <- w13
  "Accurate Data" <- w12
  "Standard Deviation of Data" <- w11
